vi "Create Coverage Report - Lines below Coverage Percentage are Hit.vi"() -> ()   [LabVIEW 2017, in "Cobertura.Tests.lvlib"]
uses:
  Cobertura.Tests.lvlib
  Fake Code Inspector/Fake Code Inspector.lvclass
  C:/Users/pasca/Projects/Home/lvunit/Cobertura/Code Inspector Base/Code Inspector Base.lvclass
  Cobertura/Coverage/Coverage.lvclass/Coverage.ctl
  Cobertura/Package/Package.lvclass/Package.ctl
  Cobertura/Class/Class.lvclass/Class.ctl
  Cobertura/Method/Method.lvclass/Method.ctl
  Cobertura/Line/Line.lvclass/Line.ctl
  Cobertura/Coverage/Read Packages.vi
  Cobertura/Package/Read Classes.vi
  Cobertura/Class/Read Methods.vi
  Cobertura/Method/Read Lines.vi
  Cobertura/Line/Read Hits.vi
  Fake Project Inspector/Fake Project Inspector.lvclass
  C:/Users/pasca/Projects/Home/lvunit/Cobertura/Project Inspector Base/Project Inspector Base.lvclass
  Fake Code Coverage/Fake Code Coverage.lvclass
  C:/Users/pasca/Projects/Home/lvunit/CodeCoverage/CodeCoverage.lvclass
  Cobertura/Package/Package.lvclass
  Cobertura/Class/Class.lvclass
  Cobertura/Method/Method.lvclass
  Cobertura/Line/Line.lvclass
  Cobertura/Cobertura.lvlib
  <vilib>/PNR/Transparent Assertions/Transparent Assertions/Transparent Assertions.lvlib
  Cobertura/Coverage/Coverage.lvclass
panel:
  out "error out":errorcluster
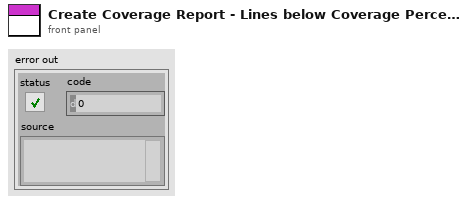
[diagram p1: front panel]
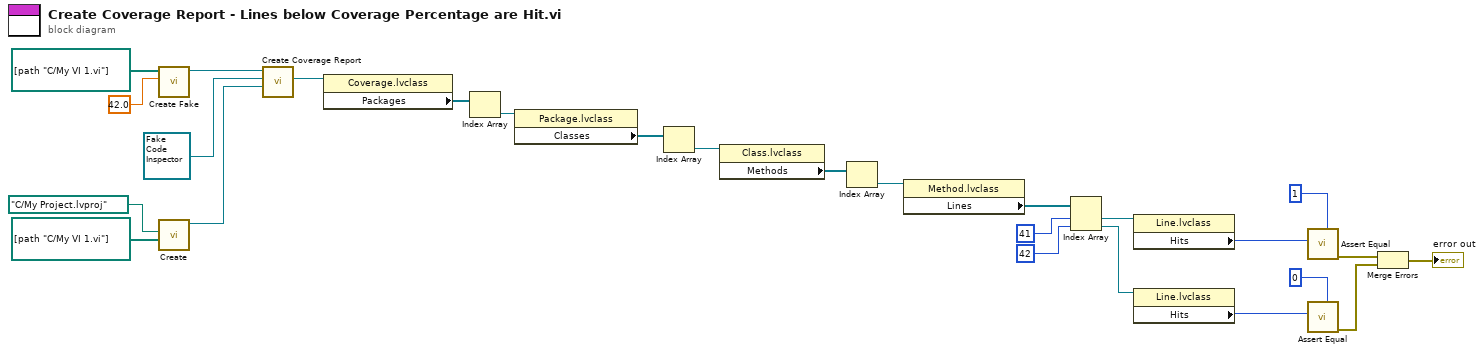
[diagram p0: block diagram]
diagram:
  n1 = call "Create Fake.vi"("Coverage Percentage"=42.0, "All VIs Measured"=path[] [path "C:/My VI 1.vi"] ("Item Paths")) -> ("Fake Code Coverage"=w16:refnum<class "Fake Code Coverage.lvclass">)  [unwired: 8 in, 1 out]
  n2 = call "Create.vi"("Item Paths"=path[] [path "C:/My VI 1.vi"], "Path"=path "C:/My Project.lvproj") -> ("Fake Project Inspector"=w24:refnum<class "Fake Project Inspector.lvclass">)  [unwired: 8 in, 1 out]
  n3 = call "Create Coverage Report.vi"("Project Inspector"=w24, "Code Inspector"=refnum<class "Fake Code Inspector.lvclass"> refnum, "CodeCoverage in"=w16) -> ("Coverage"=w26:refnum<class "Coverage.lvclass">)  [unwired: 7 in, 1 out]
  n4 = property class="Coverage.lvclass"(reference=w26) -> ("Packages"=w25:refnum<class "Package.lvclass">[])  [unwired: 1 in, 2 out]
  n5 = Index Array(array=w25) -> (element=w22:refnum<class "Package.lvclass">)  [unwired: 1 in]
  n6 = property class="Package.lvclass"(reference=w22) -> ("Classes"=w21:refnum<class "Class.lvclass">[])  [unwired: 1 in, 2 out]
  n7 = Index Array(array=w21) -> (element=w19:refnum<class "Class.lvclass">)  [unwired: 1 in]
  n8 = property class="Class.lvclass"(reference=w19) -> ("Methods"=w18:refnum<class "Method.lvclass">[])  [unwired: 1 in, 2 out]
  n9 = Index Array(array=w18) -> (element=w17:refnum<class "Method.lvclass">)  [unwired: 1 in]
  n10 = property class="Method.lvclass"(reference=w17) -> ("Lines"=w11:refnum<class "Line.lvclass">[])  [unwired: 1 in, 2 out]
  n11 = Index Array(array=w11, index #1=41 ("index"), index #2=42 ("index")) -> (element #1=w10:refnum<class "Line.lvclass">, element #2=w9:refnum<class "Line.lvclass">)
  n12 = property class="Line.lvclass"(reference=w10) -> ("Hits"=w4:u32)  [unwired: 1 in, 2 out]
  n13 = property class="Line.lvclass"(reference=w9) -> ("Hits"=w6:u32)  [unwired: 1 in, 2 out]
  n14 = call <vilib>:"Assert Equal.vi"("Expected"=u32 1 ("Branch Rate"), "Actual"=w4) -> ("error out"=w3:errorcluster)  [unwired: 9 in]
  n15 = call <vilib>:"Assert Equal.vi"("Expected"=u32 0 ("Branch Rate"), "Actual"=w6) -> ("error out"=w2:errorcluster)  [unwired: 9 in]
  n16 = Merge Errors(w3, w2) -> (→"error out":errorcluster)
